vi "KM_ControlHFLI -- V3.vi.vi"(4 "Control HFLI command":T2=enum."Scan frequency", 8 "ZI HFLI System Parameters IN":T1={"IP Address"="DEV987", "Start (Hz)"=10000.0, "Stop (Hz)"=1000000.0, "Filter Order"=4, "Number of Points"=100, "Precision"=0, "Bandwidth (Hz)"=-1.0, "Averaging"=1, "Log Sweep"=FALSE, "Demod"=3} {"Averaging" items=["1"=1, "2"=2, "4"=4, "16"=16, "32"=32, "64"=64]; "Bandwidth (Hz)" format="%#_p"; "Precision" items=["Low", "Med", "High"]; "Number of Points" min=2 max=66000; "Filter Order" items=["6, 1st"=1, "12, 2nd"=2, "18, 3rd"=3, "24, 4th"=4, "30, 5th"=5, "36, 6th"=6, "42, 7th"=7, "48, 8th"=8]; "Stop (Hz)" format="%_5p"; "Start (Hz)" format="%_5p"}) -> (0 "Voltage out":cdb[](array[numeric]), 1 "Freq out":dbl[](array[numeric]), 3 "ZI HFLI System Parameters OUT":T1={"IP Address"="DEV987", "Start (Hz)"=10000.0, "Stop (Hz)"=1000000.0, "Filter Order"=4, "Number of Points"=100, "Precision"=0, "Bandwidth (Hz)"=-1.0, "Averaging"=1, "Log Sweep"=FALSE, "Demod"=3} {"Averaging" items=["1"=1, "2"=2, "4"=4, "16"=16, "32"=32, "64"=64]; "Bandwidth (Hz)" format="%#_p"; "Precision" items=["Low", "Med", "High"]; "Number of Points" min=2 max=66000; "Filter Order" items=["6, 1st"=1, "12, 2nd"=2, "18, 3rd"=3, "24, 4th"=4, "30, 5th"=5, "36, 6th"=6, "42, 7th"=7, "48, 8th"=8]; "Stop (Hz)" format="%_5p"; "Start (Hz)" format="%_5p"})   [LabVIEW 2016]
doc: "Control a Zurich instrument device via the LabOne Labview API. \nRequirements: Zurich Instruments HF2 (HF2IS or HF2LI-MF ).\nThis example uses the API functions to perform a frequency sweep and measure the impedance. \n\n© Zurich Instruments AG, www.zhinst.com"
uses:
  <instrlib>/Zurich Instruments LabOne/Zurich Instruments LabOne.lvlib
  <instrlib>/Zurich Instruments LabOne/Public/Modules/ziTypeModEnum.ctl
  KM_ControlHFLIcommand.ctl
  KM_SystemParameters.ctl
panel:
  out "Current out":cdb[](array[numeric])
  out "Point 2":i32=10 caption="Point (#)"
  out "cal_types":cluster{string[], bool[]}[](array[cluster])=[{["R (Ohms)", " ", " "], [TRUE, FALSE, FALSE]}, {["C (F)", " ", " "], [TRUE, FALSE, FALSE]}, {["L (H)", " ", " "], [TRUE, FALSE, FALSE]}, {["R (Ohms)", "C (F)\n ", " "], [TRUE, TRUE, FALSE]}]
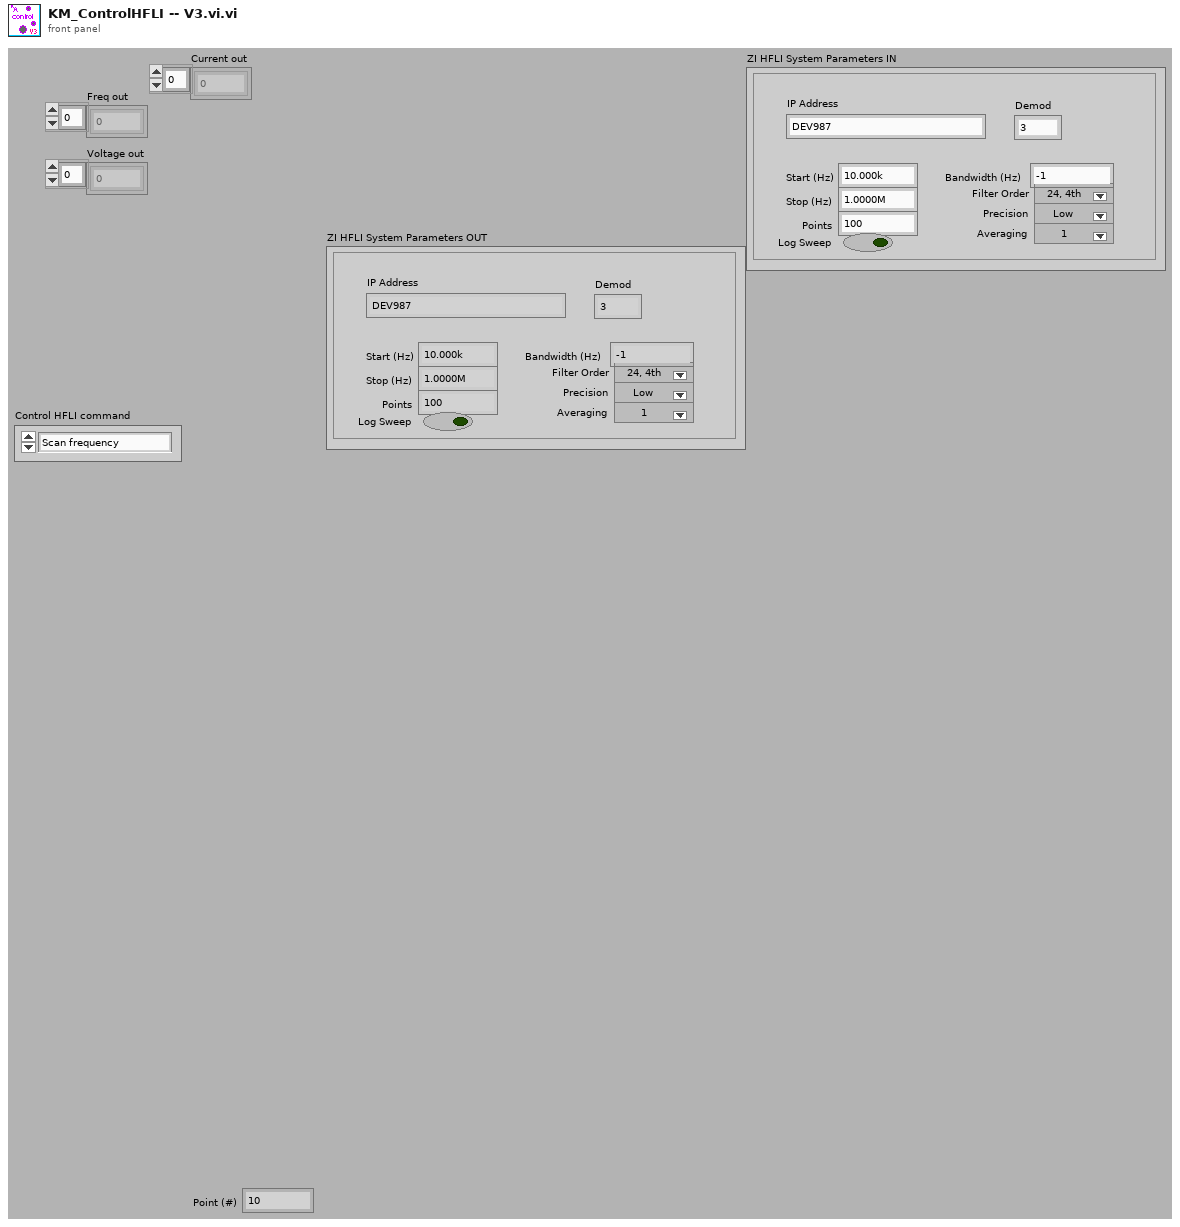
[diagram p1: front panel]
types:
  T1 = typedef "KM_SystemParameters.ctl" = cluster{"IP Address":string, "Start (Hz)":dbl, "Stop (Hz)":dbl, "Filter Order":i32, "Number of Points":i32, "Precision":u16, "Bandwidth (Hz)":dbl, "Averaging":u16, "Log Sweep":bool, "Demod":i32}
  T2 = typedef "KM_ControlHFLIcommand.ctl" = enum16{"Initialize", "Scan frequency"}
  T3 = typedef "Zurich Instruments LabOne.lvlib/ziTypeModEnum.ctl" = u16
  T4 = cluster{"Output (F,X1,Y1,X2,Y2,...,Vo)":dbl[][], "Point (#)":i32}
  T5 = typedef "Zurich Instruments LabOne.lvlib/ziTypeHandle.ctl" = cluster{"handleValid":bool, "Conn":u64, "Path Prefix":string, "Handle":u64, "Connected":bool, "Clockbase(s)":dbl}
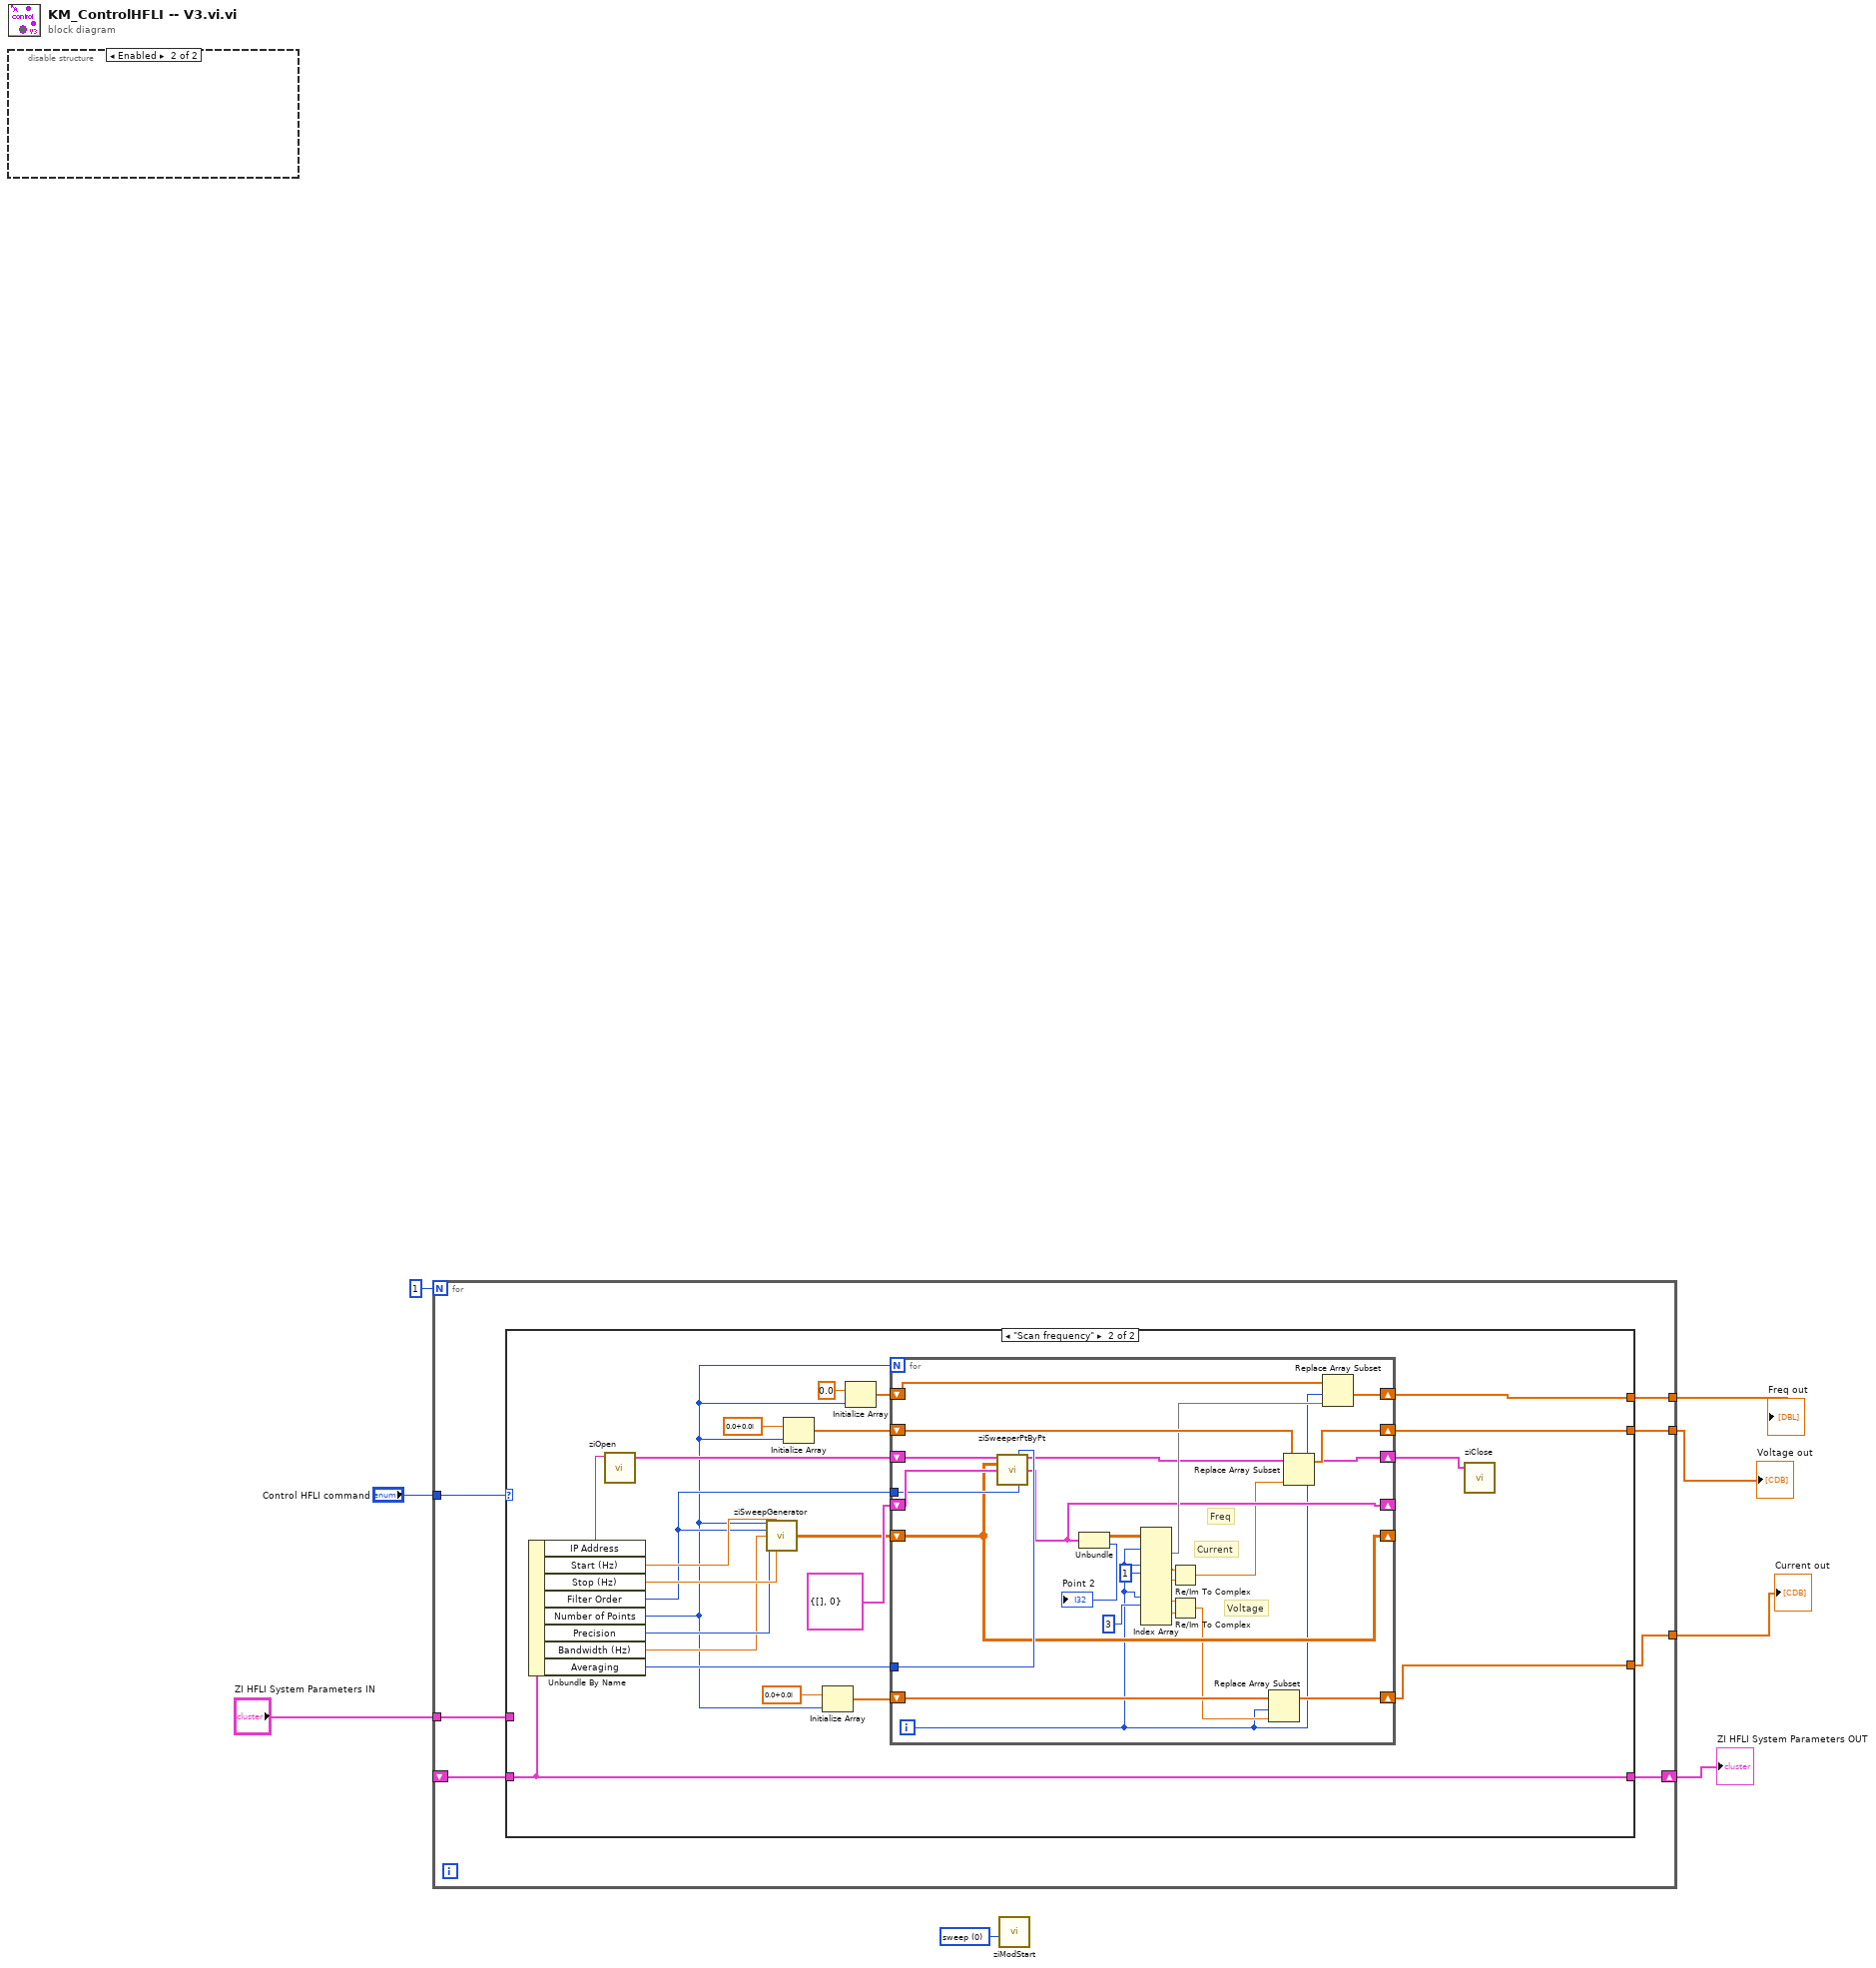
[diagram p0: block diagram]
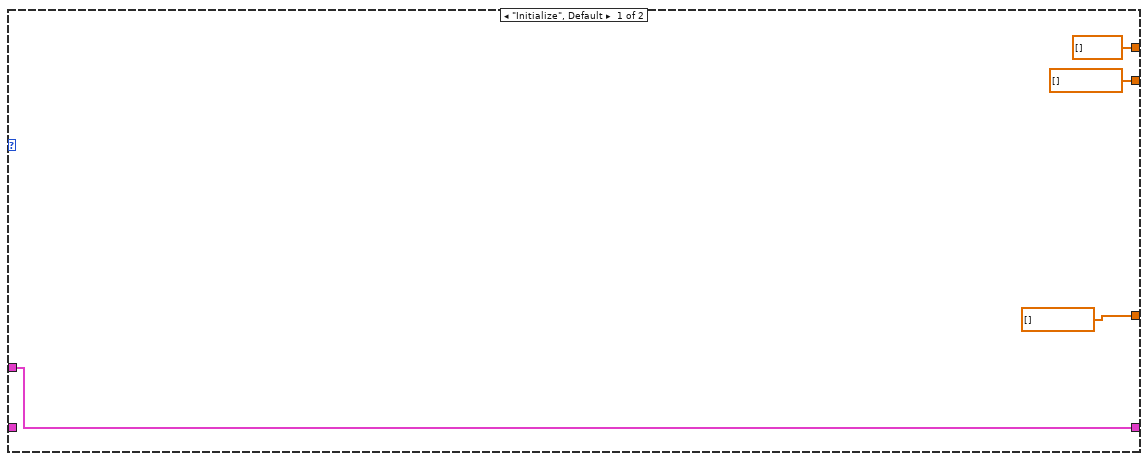
[diagram p2: hidden frame]
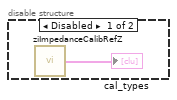
[diagram p3: hidden frame]
diagram:
  w1 = T3 0 items=["sweep", "zoomFFT", "trigger", "record", "pidAdvisor", "awgModule", "scopeModule", "impedanceModule", "multiDeviceSyncModule", "deviceSettings"] ("module Id")
  n1 = disable-structure shown="Enabled" {
    frame Disabled {
      n2 = call "ziImpedanceCalibRefZ.vi"() -> ("cal_types"=→"cal_types":cluster{string[], bool[]}[], 2:w9)  [unwired: 3 in, 1 out]
    }
    frame Enabled {
    }
  }
  n3 = for {
    N: 1 -> [_]
    tunnel: "Control HFLI command" -> [w17]
    tunnel: "ZI HFLI System Parameters IN" -> [w16]
    shift-right: [w15] -> w4
    shift-left: _ -> [w14]
    tunnel: [w13] -> w6
    tunnel: [w12] -> w5
    tunnel: [w11] -> w3
    n4 = case shown="\"Scan frequency\"" w17 {
      tunnel: w16 -> [w21 _]
      tunnel: [w21 w43] -> w15
      tunnel: w14 -> [_ w43]
      tunnel: [dbl[] [] w27] -> w13
      tunnel: [cdb[] [] w26] -> w12
      tunnel: [cdb[] [] w22] -> w11
      frame "Initialize", Default {
      }
      frame "Scan frequency" {
        n5 = Unbundle By Name(w43) -> ("IP Address"=w42:string, "Start (Hz)"=w41:dbl, "Stop (Hz)"=w40:dbl, "Filter Order"=w33:i32, "Number of Points"=w23:i32, "Precision"=w39:u16, "Bandwidth (Hz)"=w38:dbl, "Averaging"=w32:u16)
        n6 = call "ziOpen.vi"("Address"=w42) -> ("HandleOut"=w29:T5)  [unwired: 3 in, 2 out]
        n7 = call "ziSweepGenerator.vi"("Steps (#)"=w23, "Start (Hz)"=w41, "Order (4)"=w33, "Bandwith (-1=auto)"=w38, "Precision (Low)"=w39, "Stop (Hz)"=w40) -> ("Sweep Sequence (F (Hz), BW (Hz), TC(s), Time(s))"=w34:dbl[][])  [unwired: 7 in, 2 out]
        n8 = Initialize Array(cdb 0.0+0.0i ("element"), w23) -> (w36:cdb[])
        n9 = Initialize Array(cdb 0.0+0.0i ("element"), w23) -> (w24:cdb[])
        n10 = Initialize Array(0.0 ("element"), w23) -> (w30:dbl[])
        n11 = for {
          N: w23 -> [_]
          shift-right: [w67] -> w26
          shift-left: w36 -> [w68]
          shift-right: [w51] -> _
          shift-left: T4 {"Output (F,X1,Y1,X2,Y2,...,Vo)"=[], "Point (#)"=0} ("State Out") -> [w66]
          shift-right: [w52] -> _
          shift-left: w34 -> [w52]
          tunnel: w33 -> [w65]
          tunnel: w32 -> [w64]
          shift-right: [w56] -> w27
          shift-left: w30 -> [w57]
          shift-right: [w54] -> w28
          shift-left: w29 -> [w53]
          shift-right: [w46] -> w22
          shift-left: w24 -> [w47]
          i -> [w44]
          # "Voltage"
          # "Current"
          # "Freq"
          n12 = call "ziSweeperPtByPt.vi"("Handle In"=w53, "Averaging"=w64, "Sweep Sequence In"=w52, "State In"=w66, "Order (4)"=w65) -> ("Handle Out"=w54:T5, "State Out"=w51:T4)  [unwired: 7 in, 2 out]
          n13 = Unbundle(w51) -> ("Output (F,X1,Y1,X2,Y2,...,Vo)"=w58:dbl[][], "Point (#)"=→"Point 2":i32)
          n14 = Index Array(array=w58, index (row) #1=w44, index (row) #2=w44, index (col) #2=1 ("disabled index (col)"), index (row) #4=w44, index (col) #4=3 ("disabled index (col)")) -> (element #1=w55:dbl[], element #2=w62:dbl, element #3=w63:dbl, element #4=w61:dbl, element #5=w60:dbl)  [unwired: 5 in]
          n15 = Re/Im To Complex(1:w63, 2:w62) -> (0:w50:cdb)
          n16 = Re/Im To Complex(1:w60, 2:w61) -> (0:w45:cdb)
          n17 = Replace Array Subset(array=w47, new element=w45, index=w44) -> (w46:cdb[])
          n18 = Replace Array Subset(array=w68, new element=w50, index=w44) -> (w67:cdb[])
          n19 = Replace Array Subset(array=w57, new element=w55, index=w44) -> (w56:dbl[])
        }
        n20 = call "ziClose.vi"("Handle In"=w28) -> ()  [unwired: 3 in, 2 out]
      }
    }
  }
  "Freq out" <- w6
  "Voltage out" <- w5
  "ZI HFLI System Parameters OUT" <- w4
  "Current out" <- w3
  n21 = call <instrlib>:"ziModStart.vi"("module Id"=w1) -> ()  [unwired: 8 in, 3 out]
